vi "Teleop Drive.vi"(11 "Joystick Data":T1) -> ()   [LabVIEW 2013]
uses:
  Joystick Data.ctl
  Kachig.ctl
  <vilib>/Rock Robotics/WPI/RobotDrive/WPI_RobotDriveGetSetRefNum.vi
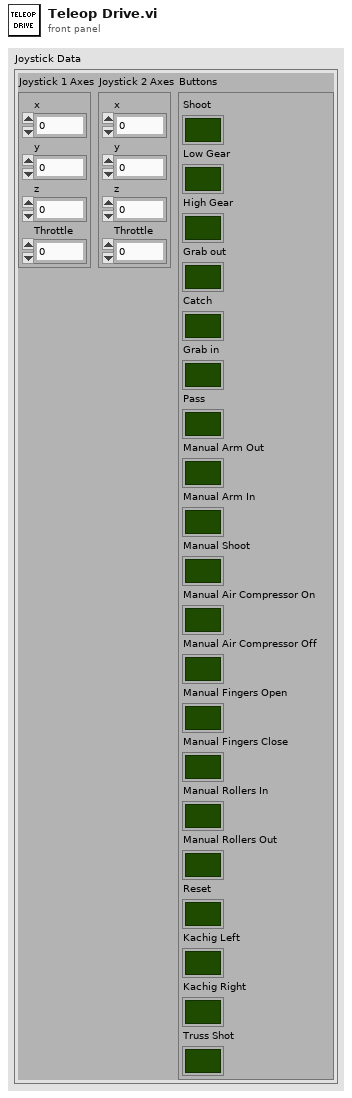
[diagram p1: front panel]
types:
  T1 = typedef "Joystick Data.ctl" = cluster{"Joystick 1 Axes":cluster{"x":dbl, "y":dbl, "z":dbl, "Throttle":dbl}, "Joystick 2 Axes":cluster{"x":dbl, "y":dbl, "z":dbl, "Throttle":dbl}, "Buttons":cluster{"Shoot":bool, "Low Gear":bool, "High Gear":bool, "Grab out":bool, "Catch":bool, "Grab in":bool, "Pass":bool, "Manual Arm Out":bool, "Manual Arm In":bool, "Manual Shoot":bool, "Manual Air Compressor On":bool, "Manual Air Compressor Off":bool, "Manual Fingers Open":bool, "Manual Fingers Close":bool, "Manual Rollers In":bool, "Manual Rollers Out":bool, "Reset":bool, "Kachig Left":bool, "Kachig Right":bool, "Truss Shot":bool}}
  T2 = typedef "Kachig.ctl" = enum16{"Idle", "Kachig Left", "Kachig Right"}
  T3 = typedef "WPI_RobotDriveDevRef.ctl" = cluster{"DevStatus":errorcluster, "Motors[]":T4[], "Square Inputs":bool, "Max Output":dbl, "Isochronous":bool}
  T4 = typedef "WPI_MotorControlDeviceRef.ctl" = cluster{"DeviceStatus":errorcluster, "Type":enum16{"PWM", "CAN"}, "PWM":cluster{"Digital Module":T5, "PWM Channel":T6, "DeadBand":T7}, "CAN":cluster{"Device Number":u8, "Control Mode":T8, "Semaphore":T9, "Max Vout":dbl}, "Invert":bool, "TransformRef":T10, "InvTransformRef":T10}
  T5 = typedef "FPGA_TypedefDigitalModule.ctl" = enum16{"Digital Module 1", "Digital Module 2"}
  T6 = typedef "FPGA_DIOPWMChannel.ctl" = enum8{"PWM 1", "PWM 2", "PWM 3", "PWM 4", "PWM 5", "PWM 6", "PWM 7", "PWM 8", "PWM 9", "PWM 10", "Invalid"}
  T7 = typedef "WPI_PWMDeadband.ctl" = cluster{"Name":string, "maxPositivePwm":i32, "minPositivePwm":i32, "centerPwm":i32, "maxNegativePwm":i32, "minNegativePwm":i32, "angularRange":u16}
  T8 = typedef "WPI_CANJaguar_ControlMode.ctl" = enum8{"Percent VBus", "Current", "Speed", "Position", "Voltage"}
  T9 = typedef "Semaphore RefNum" = refnum<k1>
  T10 = typedef "WPI_PWMTransform_ConPane.ctl" = refnum<vi>
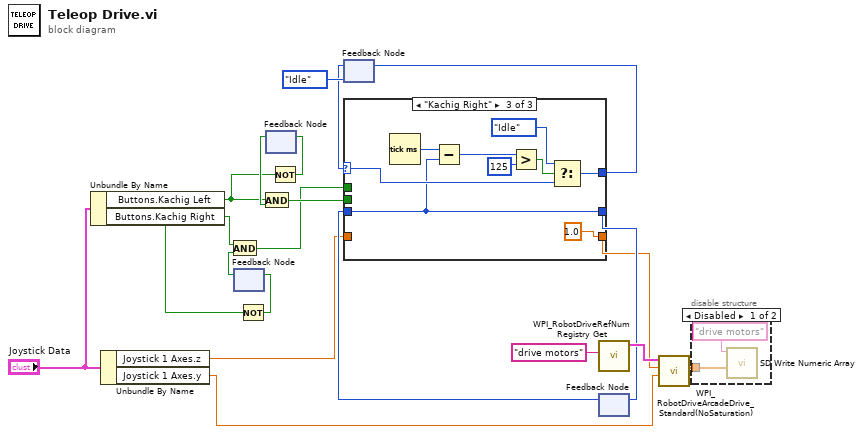
[diagram p0: block diagram]
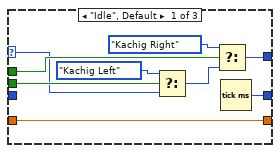
[diagram p3: hidden frame]
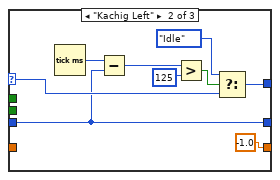
[diagram p4: hidden frame]
diagram:
  n1 = Unbundle By Name("Joystick Data") -> ("Buttons.Kachig Left"=w7:bool, "Buttons.Kachig Right"=w3:bool)
  n2 = Unbundle By Name("Joystick Data") -> ("Joystick 1 Axes.z"=w9:dbl, "Joystick 1 Axes.y"=w17:dbl)
  n3 = feedback #1() -> (w4:bool)  [unwired: 1 in]
  n4 = And(x=w3, y=w4) -> (x .and. y?=w1:bool)
  n5 = Not(x=w3) -> (.not. x?=w2:bool)
  n6 = feedback-in #1(w2) -> ()
  n7 = feedback #2() -> (w8:bool)  [unwired: 1 in]
  n8 = And(x=w7, y=w8) -> (x .and. y?=w5:bool)
  n9 = Not(x=w7) -> (.not. x?=w6:bool)
  n10 = feedback-in #2(w6) -> ()
  n11 = feedback #3(Kachig."Idle") -> (w14:T2)
  n12 = call <vilib>:"WPI_RobotDriveRefNum Registry Get.vi"("refnum name"="drive motors") -> ("RobotDriveDevRef"=w19:T3)  [unwired: 1 in, 9 out]
  n13 = feedback #4() -> (w12:u32)  [unwired: 1 in]
  n14 = case shown="\"Kachig Right\"" w14 {
    selector: w14 -> [w24 w31 w41]
    tunnel: [w23 w30 w40] -> w13
    tunnel: w12 -> [_ w30 w40]
    tunnel: w5 -> [w29 _ _]
    tunnel: w1 -> [w28 _ _]
    tunnel: [w22 w35 w39] -> w11
    tunnel: [w21 -1.0 1.0] -> w10
    tunnel: w9 -> [w21 _ _]
    frame "Idle", Default {
      n15 = Select(t=Kachig."Kachig Left", s=w29, f=w24) -> (s? t:f=w27:T2)
      n16 = Select(t=Kachig."Kachig Right", s=w28, f=w27) -> (s? t:f=w22:T2)
      n17 = Tick Count (ms)() -> (millisecond timer value=w23:u32)
    }
    frame "Kachig Left" {
      n18 = Tick Count (ms)() -> (millisecond timer value=w34:u32)
      n19 = Subtract(x=w34, y=w30) -> (x-y=w37:u32)
      n20 = Greater?(x=w37, y=125) -> (0:w36:bool)
      n21 = Select(t=Kachig."Idle", s=w36, f=w31) -> (s? t:f=w35:T2)
    }
    frame "Kachig Right" {
      n22 = Tick Count (ms)() -> (millisecond timer value=w44:u32)
      n23 = Subtract(x=w44, y=w40) -> (x-y=w42:u32)
      n24 = Greater?(x=w42, y=125) -> (0:w43:bool)
      n25 = Select(t=Kachig."Idle", s=w43, f=w41) -> (s? t:f=w39:T2)
    }
  }
  n26 = feedback-in #3(w11) -> ()
  n27 = feedback-in #4(w13) -> ()
  n28 = call <vilib>:"WPI_RobotDriveArcadeDrive_Standard(NoSaturation).vi"("Y axis value"=w17, "X axis value"=w10, "RobotDriveDevRef"=w19) -> ("Motor Values"=w20:dbl[])  [unwired: 1 in, 7 out]
  n29 = disable-structure shown="Disabled" {
    disable-tunnel: w20 -> [w49 _]
    frame Disabled {
      n30 = call <vilib>:"SD Write Numeric Array.vi"("Numeric Array"=w49, "Name"="drive motors") -> ()  [unwired: 8 in, 2 out]
    }
    frame Enabled {
    }
  }
